vi "Set Analogical to Digital Channel.vi"(8 "error in (no error)":errorcluster, 11 "CCDCamera in":refnum<class "CCDCamera.lvclass">) -> (0 "error out":errorcluster, 3 "CCDCamera out":refnum<class "CCDCamera.lvclass">)   [LabVIEW 2018, in "CCDCamera.lvclass"]
uses:
  CCDCamera.lvclass
  Simulated_CCD_Camera/Simulated_CCD_Camera.lvclass
  Interface/Interface.lvclass
  C:/Users/observer/Desktop/SPARC4_ACS/SPARC4_ACS/Simulated_CCD_Camera/Simulated_CCD_Camera.lvclass
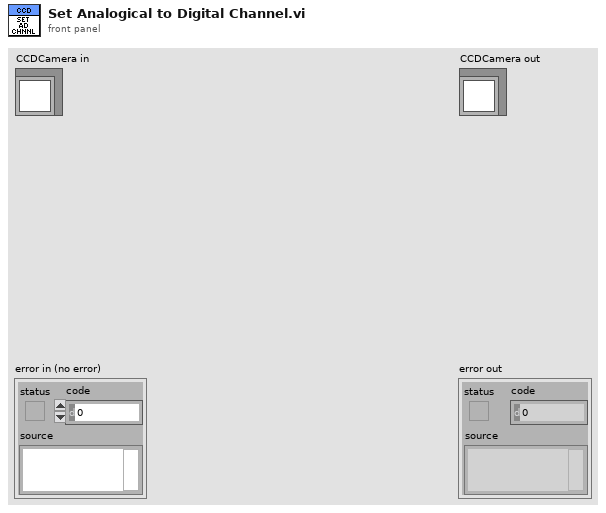
[diagram p1: front panel]
types:
  T1 = typedef "Shutter_mode typedef.ctl" = enum16{"Auto", "Open", "Close", "N/A (3)", "Open FVB Series", "Open Any Series"}
  T2 = typedef "ReadMode_mode typedef.ctl" = enum16{"Full Vertical Binning", "Multi-Track", "Random-Track", "Single-Track", "Image"}
  T3 = typedef "AcquisitionMode_mode typedef.ctl" = enum16{"Reserved (0)", "Single Scan", "Accumulate", "Kinetics", "Fast Kinetics", "Run Till Abort", "Reserved (6)", "Reserved (7)", "Reserved (8)", "Time Delayed Integration"}
  T4 = cluster{"EXPTIME":sgl, "PREAMP":enum16{"Gain 1", "Gain 2"}, "READOUT_RATE":enum16{"30 MHz", "20 MHz", "10 MHz", "1 MHz"}, "EM_GAIN":u16, "VBIN":u16, "INITIAL_LINE":u16, "INITIAL_COLUMN":u16, "FINAL_LINE":u16, "FINAL_COLUMN":u16, "#FRAMES":u32, "#CUBES":u32, "TRIGGER_MODE":enum16{"Internal", "External", "N/A", "N/A_1", "N/A_2", "N/A_3", "External Start"}, "HBIN":u16, "SHUTTER_TTL":enum16{"TTL Low", "TTL High"}, "SHUTTER_MODE":T1, "SHUTTER_OPENING_TIME":u16, "SHUTTER_CLOSING_TIME":u16, "VERTICAL_SHIFT_SPEED":u16, "READ_MODE":T2, "FRAME_TRANSFER":bool, "VERTICAL_CLOCK_VOLTAGE":enum16{"0", "+1", "+2", "+3", "+4"}, "ACQUISITION_MODE":T3, "AD_CHANNEL":u16, "EM_MODE":enum16{"Electron Multiplying", "Conventional"}}
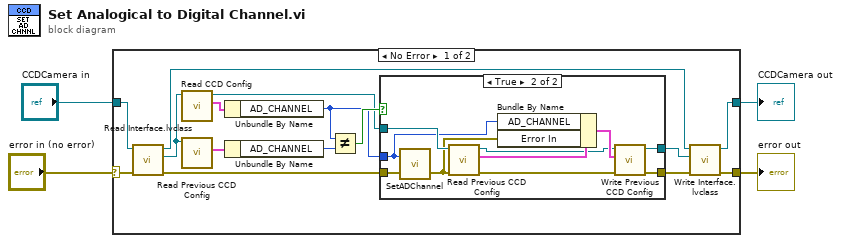
[diagram p0: block diagram]
diagram:
  n1 = case shown="No Error" "error in (no error)" {
    selector: "error in (no error)" -> [w18 w33]
    tunnel: [w6 w33] -> w3
    tunnel: [w7 w32] -> w1
    tunnel: "CCDCamera in" -> [w19 w32]
    frame No Error {
      n2 = call "Read Interface.lvclass.vi"("error in (no error)"=w18, "Simulated_CCD_Camera in"=w19) -> ("error out"=w11:errorcluster, "Interface.lvclass"=w17:refnum<class "Interface.lvclass">, "Simulated_CCD_Camera out"=w8:refnum<class "CCDCamera.lvclass">)  [unwired: 7 in]
      n3 = call "Read CCD Config.vi"("Interface in"=w17) -> ("CCD Config"=w16:T4, "Interface out"=w12:refnum<class "Interface.lvclass">)  [unwired: 8 in, 1 out]
      n4 = call "Read Previous CCD Config.vi"("Interface in"=w17) -> ("Previous CCD Config"=w15:T4)  [unwired: 8 in, 2 out]
      n5 = Unbundle By Name(w16) -> ("AD_CHANNEL"=w5:u16)
      n6 = Unbundle By Name(w15) -> ("AD_CHANNEL"=w14:u16)
      n7 = Not Equal?(x=w5, y=w14) -> (x != y?=w13:bool)
      n8 = case shown="True" w13 {
        tunnel: w12 -> [w21 w31]
        tunnel: w11 -> [w20 w23]
        tunnel: [w21 w26] -> w10
        tunnel: [w20 w25] -> w9
        tunnel: w5 -> [_ w22]
        frame False {
        }
        frame True {
          n9 = call <userlib>:"SetADChannel.vi"("error in (no error)"=w23, "channel"=w22) -> ("error out"=w24:errorcluster)  [unwired: 1 out]
          n10 = call "Read Previous CCD Config.vi"("error in (no error)"=w24, "Interface in"=w31) -> ("error out"=w28:errorcluster, "Previous CCD Config"=w30:T4, "Interface out"=w27:refnum<class "Interface.lvclass">)  [unwired: 7 in]
          n11 = Bundle By Name(cluster=w30, "AD_CHANNEL"=w22, "Error In"=w24) -> (w29:T4)
          n12 = call "Write Previous CCD Config.vi"("error in (no error)"=w28, "Previous CCD Config"=w29, "Interface in"=w27) -> ("error out"=w25:errorcluster, "Interface out"=w26:refnum<class "Interface.lvclass">)  [unwired: 7 in]
        }
      }
      n13 = call "Write Interface.lvclass.vi"("error in (no error)"=w9, "Interface.lvclass"=w10, "Simulated_CCD_Camera in"=w8) -> ("error out"=w6:errorcluster, "Simulated_CCD_Camera out"=w7:refnum<class "CCDCamera.lvclass">)  [unwired: 7 in]
    }
    frame Error {
    }
  }
  "error out" <- w3
  "CCDCamera out" <- w1
